vi "VMI_save_IF32_path.vi"(3 "Analysis Path":path) -> (0 "cancelled":bool, 1 "selected path":path)   [LabVIEW 2018]
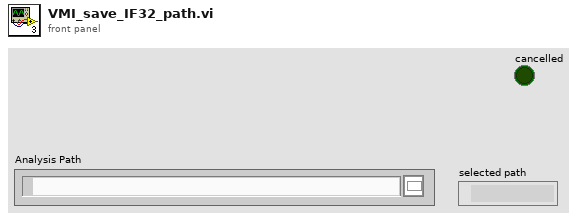
[diagram p1: front panel]
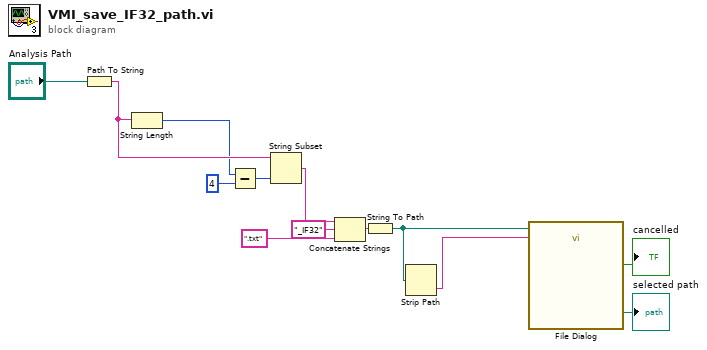
[diagram p0: block diagram]
diagram:
  n1 = Path To String(path="Analysis Path") -> (string=w12:string)
  n2 = String Length(string=w12) -> (length=w10:i32)
  n3 = Subtract(x=w10, y=4) -> (x-y=w11:i32)
  n4 = String Subset(string=w12, length (rest)=w11) -> (substring=w8:string)  [unwired: 1 in]
  n5 = Concatenate Strings(w8, "_IF32" ("string"), ".txt" ("string")) -> (w5:string)
  n6 = String To Path(string=w5) -> (path=w4:path)
  n7 = Strip Path(path=w4) -> (name=w3:string)  [unwired: 1 out]
  n8 = call "File Dialog"("start path"=w4, "default name"=w3) -> ("selected path"=→"selected path":path, "cancelled"=→"cancelled":bool)  [unwired: 10 in, 2 out]
